vi "CalculateFeatures.vi"(7 "channels":T4[](array[typedef]), 8 "error in (no error)":errorcluster, 9 "pulse positions array":T3[](array[typedef]), 10 "waveforms":T2, 11 "Map":T1) -> (0 "error out":errorcluster, 5 "channels out":T4[](array[typedef]))   [LabVIEW 2017, in "AnalysisHelper.lvlib"]
uses:
  <vilib>/addons/InsightCM/Utilities/Analysis/Shared/AnalysisHelper.lvlib
  <vilib>/addons/InsightCM/Utilities/Analysis/Shared/controls/Channel.ctl
  <vilib>/addons/InsightCM/Utilities/Analysis/Shared/controls/SpeedType.ctl
  <vilib>/addons/InsightCM/Utilities/Analysis/Shared/controls/Feature.ctl
  <vilib>/addons/InsightCM/Utilities/Analysis/Shared/controls/AmplitudeScale.ctl
  <vilib>/addons/InsightCM/Utilities/Analysis/Shared/controls/PulsePositions.ctl
  <vilib>/addons/InsightCM/Utilities/DataAccessors/controls/wfmSGL_DVR.ctl
  <vilib>/addons/PointValueMap/controls/PointMap.ctl
  <vilib>/addons/InsightCM/Utilities/ChannelStatus/ChannelStatus.lvlib
  <vilib>/addons/PointValueMap/PointValueMap.lvlib
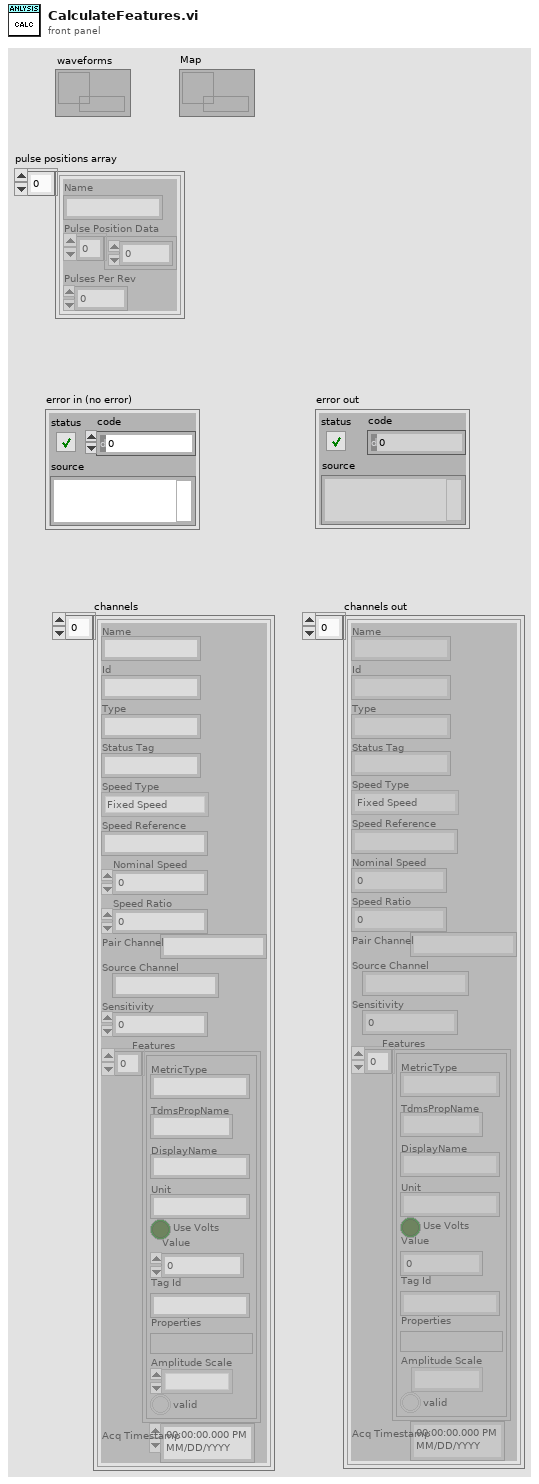
[diagram p1: front panel]
types:
  T1 = typedef "PointValueMap.lvlib/PointMap.ctl" = refnum<data-value>
  T2 = typedef "wfmSGL_DVR.ctl" = refnum<data-value>
  T3 = typedef "AnalysisHelper.lvlib/PulsePositions.ctl" = cluster{"Name":string, "Pulse Position Data":dbl[], "Pulses Per Rev":i32}
  T4 = typedef "AnalysisHelper.lvlib/Channel.ctl" = cluster{"Name":string, "Id":string, "Type":string, "Status Tag":string, "Speed Type":T5, "Speed Reference":string, "Nominal Speed":dbl, "Speed Ratio":dbl, "Pair Channel":string, "Source Channel":string, "Sensitivity":dbl, "Features":T6[], "Acq Timestamp":timestamp}
  T5 = typedef "AnalysisHelper.lvlib/SpeedType.ctl" = enum16{"Fixed Speed", "Tachometer", "From Map"}
  T6 = typedef "AnalysisHelper.lvlib/Feature.ctl" = cluster{"MetricType":string, "TdmsPropName":string, "DisplayName":string, "Unit":string, "Use Volts":bool, "Value":dbl, "Tag Id":string, "Properties":variant, "Amplitude Scale":T7, "valid":bool}
  T7 = typedef "AnalysisHelper.lvlib/AmplitudeScale.ctl" = enum16{"rms", "peak", "pk-pk"}
  T8 = typedef "AnalysisHelper.lvlib/LevelFeatures.ctl" = cluster{"RMS":dbl, "Peak":dbl, "Pk-Pk":dbl, "Derived Peak":dbl, "Crest Factor":dbl}
  T9 = typedef "AnalysisHelper.lvlib/MaxMinAvgFeatures.ctl" = cluster{"Max":dbl, "Min":dbl, "Avg":dbl}
  T10 = typedef "AnalysisHelper.lvlib/ConversionOp.ctl" = enum16{"none", "singleInt", "doubleInt", "singleDiff", "doubleDiff"}
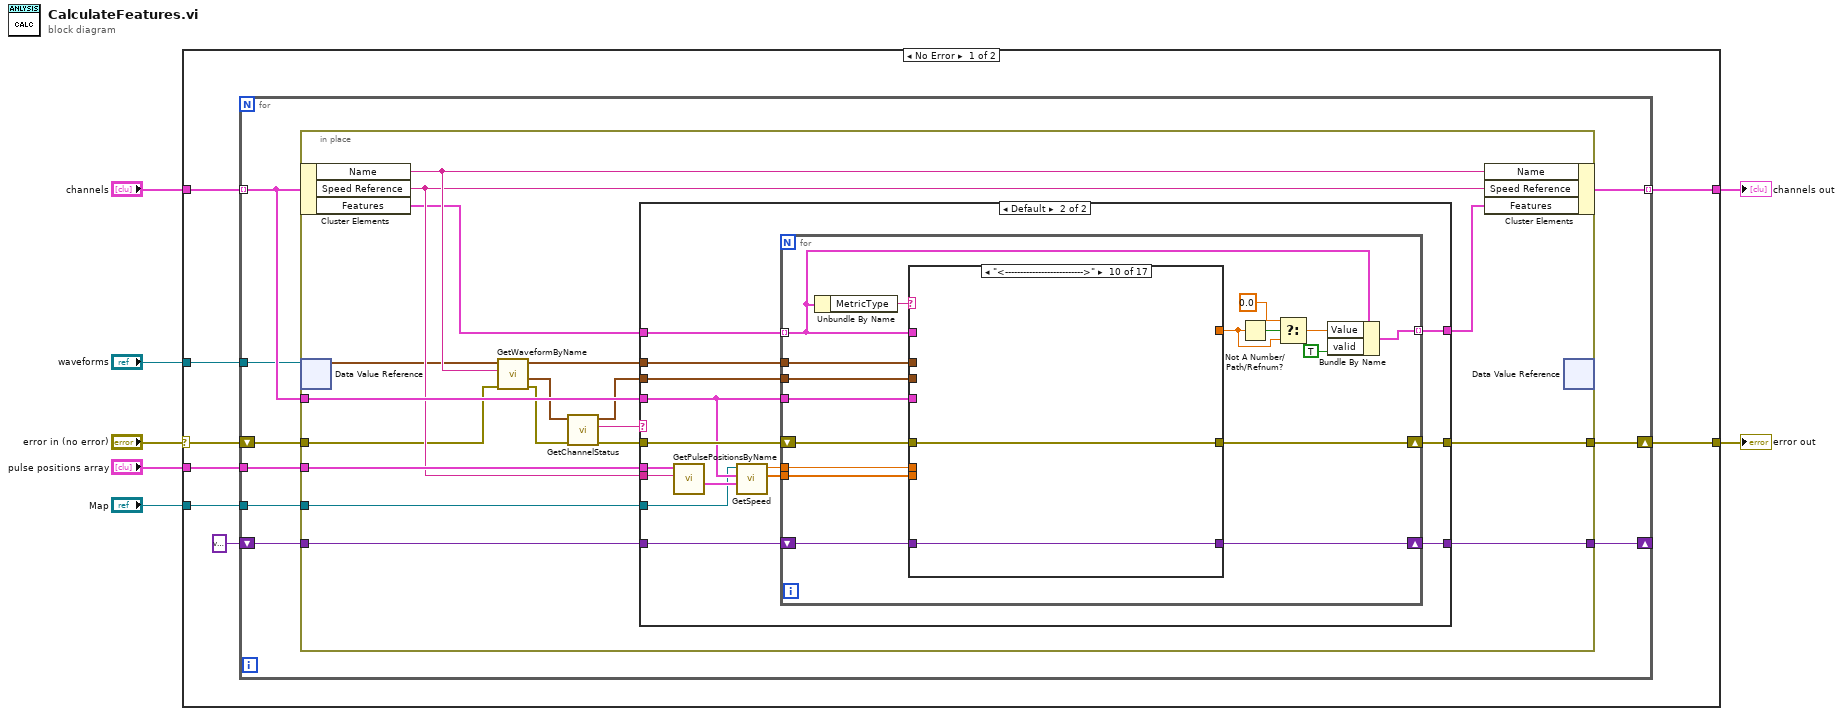
[diagram p0: block diagram]
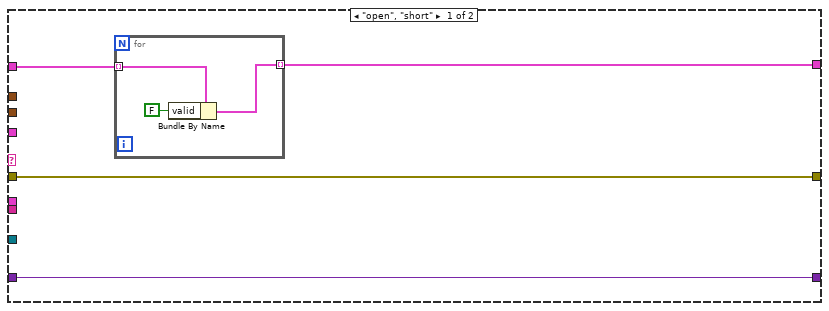
[diagram p2: hidden frame]
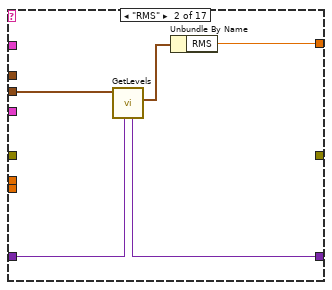
[diagram p4: hidden frame]
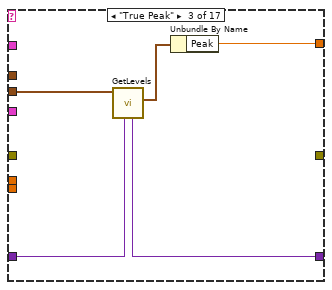
[diagram p5: hidden frame]
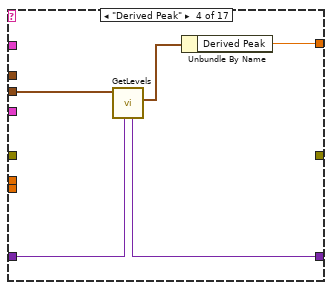
[diagram p6: hidden frame]
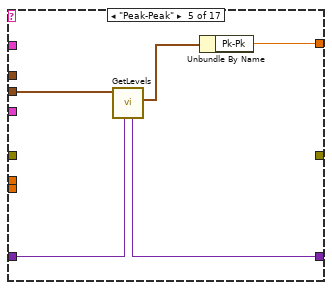
[diagram p7: hidden frame]
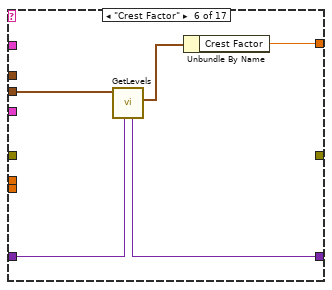
[diagram p8: hidden frame]
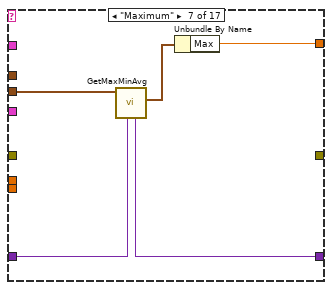
[diagram p9: hidden frame]
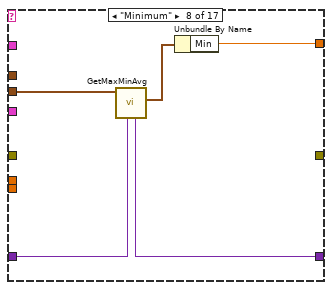
[diagram p10: hidden frame]
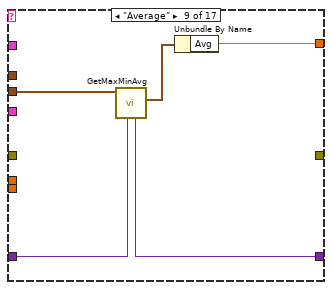
[diagram p11: hidden frame]
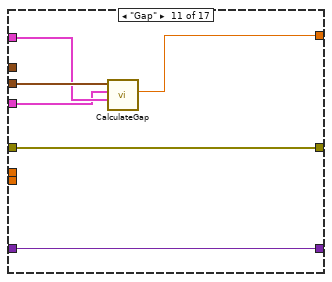
[diagram p12: hidden frame]
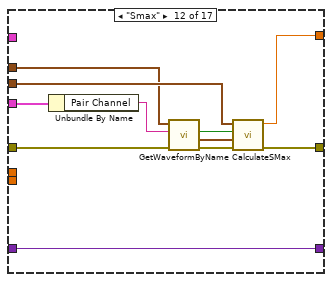
[diagram p13: hidden frame]
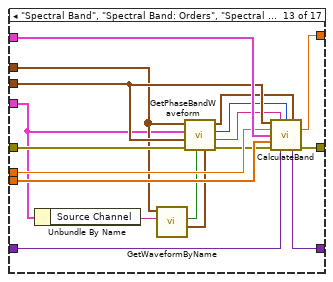
[diagram p14: hidden frame]
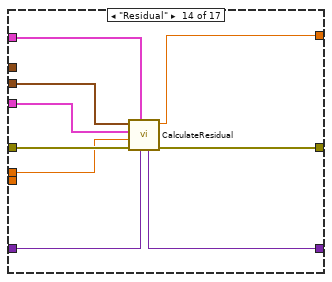
[diagram p15: hidden frame]
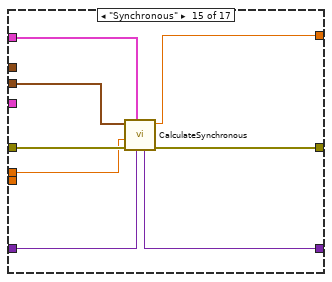
[diagram p16: hidden frame]
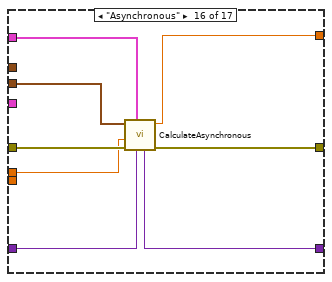
[diagram p17: hidden frame]
diagram:
  n1 = case shown="No Error" "error in (no error)" {
    selector: "error in (no error)" -> [w15 w188]
    tunnel: [w10 w188] -> w7
    tunnel: "channels" -> [w13 w189]
    tunnel: [w14 w189] -> w6
    tunnel: "pulse positions array" -> [w12 _]
    tunnel: "waveforms" -> [w9 _]
    tunnel: "Map" -> [w8 _]
    frame No Error {
      n2 = for {
        tunnel: w13 -> [w21] mode=indexing
        tunnel: [w24] -> w14 mode=indexing
        tunnel: w12 -> [w20]
        shift-right: [w18] -> _
        shift-left: variant -> [w19]
        shift-right: [w22] -> w10
        shift-left: w15 -> [w23]
        tunnel: w9 -> [w17]
        tunnel: w8 -> [w16]
        n3 = in-place {
          in-place-border: w23 -> [w34]
          in-place-border: [w42] -> w22
          in-place-border: w21 -> [w40]
          in-place-border: w20 -> [w37]
          in-place-border: w19 -> [w39]
          in-place-border: [w38] -> w18
          in-place-border: w16 -> [w25]
          n4 = in-place-cluster #1(w21) -> ("Name"=w41:string, "Speed Reference"=w35:string, "Features"=w33:T6[])
          n5 = in-place-dvr #2(w17) -> (w26:waveform(sgl)[])  [unwired: 1 out]
          n6 = call <vilib>:"GetWaveformByName.vi"("error in (no error)"=w34, "Channel Name"=w41, "Acq Waveforms"=w26) -> ("error out"=w31:errorcluster, "Waveform"=w28:waveform(sgl), "Acq Waveforms Out"=w36:waveform(sgl)[])  [unwired: 5 in, 1 out]
          n7 = call <vilib>:"GetChannelStatus.vi"("error in (no error)"=w31, "waveform in"=w28) -> ("error out"=w30:errorcluster, "channel status"=w29:string, "waveform out"=w27:waveform(sgl))  [unwired: 6 in, 1 out]
          n8 = case shown="Default" w29 {
            tunnel: [w44 w64] -> w32
            tunnel: w30 -> [w43 w63]
            tunnel: w33 -> [w45 w62]
            tunnel: w40 -> [_ w53]
            tunnel: w36 -> [_ w61]
            tunnel: w27 -> [_ w60]
            tunnel: [w43 w57] -> w42
            tunnel: w39 -> [w46 w59]
            tunnel: [w46 w58] -> w38
            tunnel: w37 -> [_ w56]
            tunnel: w35 -> [_ w55]
            tunnel: w25 -> [_ w50]
            frame "open", "short" {
              n9 = for {
                tunnel: w45 -> [w49] mode=indexing
                tunnel: [w47] -> w44 mode=indexing
                n10 = Bundle By Name(cluster=w49, "valid"=FALSE) -> (w47:T6)
              }
            }
            frame Default {
              n11 = call <vilib>:"GetPulsePositionsByName.vi"("Channel Name"=w55, "Pulse Positions Array"=w56) -> ("Pulse Positions"=w54:T3)  [unwired: 6 in, 3 out]
              n12 = call <vilib>:"GetSpeed.vi"("pulse positions"=w54, "channel"=w53, "Map"=w50) -> ("pulse position data"=w52:dbl[], "speed (RPM)"=w51:dbl)  [unwired: 7 in]
              n13 = for {
                tunnel: w62 -> [w75] mode=indexing
                tunnel: w60 -> [w80]
                tunnel: [w81] -> w64 mode=indexing
                tunnel: w61 -> [w77]
                tunnel: w53 -> [w76]
                shift-right: [w72] -> w58
                shift-left: w59 -> [w73]
                shift-right: [w78] -> w57
                shift-left: w63 -> [w79]
                tunnel: w52 -> [w70]
                tunnel: w51 -> [w71]
                n14 = Unbundle By Name(w75) -> ("MetricType"=w74:string)
                n15 = case shown="\"<-------------------------->\"" w74 {
                  tunnel: [w82 w84 w89 w94 w99 w104 w111 w116 w121 _ w130 w141 w159 w166 w171 w178 _] -> w67
                  tunnel: w80 -> [_ w87 w92 w97 w102 w107 w112 w117 w122 _ w131 w140 w153 w168 w177 w184 _]
                  tunnel: w79 -> [_ _ _ _ _ _ _ _ _ w124 w129 w135 w152 w169 w176 w183 w186]
                  tunnel: [_ _ _ _ _ _ _ _ _ w124 w129 w142 w160 w167 w175 w182 w186] -> w78
                  tunnel: w77 -> [_ _ _ _ _ _ _ _ _ _ _ w136 w147 _ _ _ _]
                  tunnel: w76 -> [_ _ _ _ _ _ _ _ _ _ w127 w137 w146 w165 _ _ _]
                  tunnel: w75 -> [_ _ _ _ _ _ _ _ _ _ w128 _ w158 w164 w170 w185 _]
                  tunnel: w73 -> [w83 w86 w91 w96 w101 w106 w110 w115 w120 w125 w126 w139 w156 w162 w174 w181 w187]
                  tunnel: [w83 w85 w90 w95 w100 w105 w109 w114 w119 w125 w126 w139 w157 w163 w173 w180 w187] -> w72
                  tunnel: w71 -> [w82 _ _ _ _ _ _ _ _ _ _ _ w154 w161 w172 w179 _]
                  tunnel: w70 -> [_ _ _ _ _ _ _ _ _ _ _ _ w155 _ _ _ _]
                  frame "Speed" {
                  }
                  frame "RMS" {
                    n16 = call <vilib>:"GetLevels.vi"("calc cache"=w86, "waveform"=w87) -> ("levels"=w88:T8, "calc cache out"=w85:variant)  [unwired: 8 in]
                    n17 = Unbundle By Name(w88) -> ("RMS"=w84:dbl)
                  }
                  frame "True Peak" {
                    n18 = call <vilib>:"GetLevels.vi"("calc cache"=w91, "waveform"=w92) -> ("levels"=w93:T8, "calc cache out"=w90:variant)  [unwired: 8 in]
                    n19 = Unbundle By Name(w93) -> ("Peak"=w89:dbl)
                  }
                  frame "Derived Peak" {
                    n20 = call <vilib>:"GetLevels.vi"("calc cache"=w96, "waveform"=w97) -> ("levels"=w98:T8, "calc cache out"=w95:variant)  [unwired: 8 in]
                    n21 = Unbundle By Name(w98) -> ("Derived Peak"=w94:dbl)
                  }
                  frame "Peak-Peak" {
                    n22 = call <vilib>:"GetLevels.vi"("calc cache"=w101, "waveform"=w102) -> ("levels"=w103:T8, "calc cache out"=w100:variant)  [unwired: 8 in]
                    n23 = Unbundle By Name(w103) -> ("Pk-Pk"=w99:dbl)
                  }
                  frame "Crest Factor" {
                    n24 = call <vilib>:"GetLevels.vi"("calc cache"=w106, "waveform"=w107) -> ("levels"=w108:T8, "calc cache out"=w105:variant)  [unwired: 8 in]
                    n25 = Unbundle By Name(w108) -> ("Crest Factor"=w104:dbl)
                  }
                  frame "Maximum" {
                    n26 = call <vilib>:"GetMaxMinAvg.vi"("calc cache"=w110, "waveform"=w112) -> ("MaxMinAvg"=w113:T9, "calc cache out"=w109:variant)  [unwired: 8 in]
                    n27 = Unbundle By Name(w113) -> ("Max"=w111:dbl)
                  }
                  frame "Minimum" {
                    n28 = call <vilib>:"GetMaxMinAvg.vi"("calc cache"=w115, "waveform"=w117) -> ("MaxMinAvg"=w118:T9, "calc cache out"=w114:variant)  [unwired: 8 in]
                    n29 = Unbundle By Name(w118) -> ("Min"=w116:dbl)
                  }
                  frame "Average" {
                    n30 = call <vilib>:"GetMaxMinAvg.vi"("calc cache"=w120, "waveform"=w122) -> ("MaxMinAvg"=w123:T9, "calc cache out"=w119:variant)  [unwired: 8 in]
                    n31 = Unbundle By Name(w123) -> ("Avg"=w121:dbl)
                  }
                  frame "<-------------------------->" {
                  }
                  frame "Gap" {
                    n32 = call <vilib>:"CalculateGap.vi"("feature"=w128, "channel"=w127, "waveform data"=w131) -> ("gap"=w130:dbl)  [unwired: 8 in]
                  }
                  frame "Smax" {
                    n33 = Unbundle By Name(w137) -> ("Pair Channel"=w138:string)
                    n34 = call <vilib>:"GetWaveformByName.vi"("error in (no error)"=w135, "Channel Name"=w138, "Acq Waveforms"=w136) -> ("error out"=w134:errorcluster, "Waveform"=w132:waveform(sgl), "Found?"=w133:bool)  [unwired: 5 in, 1 out]
                    n35 = call <vilib>:"CalculateSMax.vi"("error in (no error)"=w134, "pair waveform"=w132, "pair waveform found"=w133, "Waveform"=w140) -> ("error out"=w142:errorcluster, "Smax"=w141:dbl)  [unwired: 6 in]
                  }
                  frame "Spectral Band", "Spectral Band: Orders", "Spectral Band: Phase" {
                    n36 = Unbundle By Name(w146) -> ("Source Channel"=w145:string)
                    n37 = call <vilib>:"GetWaveformByName.vi"("Channel Name"=w145, "Acq Waveforms"=w147) -> ("Waveform"=w143:waveform(sgl), "Found?"=w144:bool)  [unwired: 6 in, 2 out]
                    n38 = call <vilib>:"GetPhaseBandWaveform.vi"("source channel wfm"=w143, "source channel wfm found"=w144, "error in (no error)"=w152, "waveform"=w153, "channel"=w146, "all waveforms"=w147) -> ("error out"=w151:errorcluster, "channel name of waveform to use in phase band calculation"=w148:string, "conversion op"=w149:T10, "waveform to use in phase band calculation"=w150:waveform(sgl))  [unwired: 2 in]
                    n39 = call <vilib>:"CalculateBand.vi"("waveform"=w153, "channel name of waveform to use in phase band calculation"=w148, "conversion op"=w149, "waveform to use in phase band calculation"=w150, "speed [RPM]"=w154, "feature"=w158, "pulse positions"=w155, "error in (no error)"=w151, "calc cache"=w156) -> ("band value"=w159:dbl, "calc cache out"=w157:variant, "error out"=w160:errorcluster)  [unwired: 4 in]
                  }
                  frame "Residual" {
                    n40 = call <vilib>:"CalculateResidual.vi"("calc cache"=w162, "Feature"=w164, "error in (no error)"=w169, "Speed (RPM)"=w161, "Channel"=w165, "Data"=w168) -> ("error out"=w167:errorcluster, "Residual [EU RMS]"=w166:dbl, "calc cache out"=w163:variant)  [unwired: 3 in]
                  }
                  frame "Synchronous" {
                    n41 = call <vilib>:"CalculateSynchronous.vi"("calc cache"=w174, "Feature"=w170, "error in (no error)"=w176, "Speed (RPM)"=w172, "Data"=w177) -> ("error out"=w175:errorcluster, "Synchronous [EU RMS]"=w171:dbl, "calc cache out"=w173:variant)  [unwired: 4 in]
                  }
                  frame "Asynchronous" {
                    n42 = call <vilib>:"CalculateAsynchronous.vi"("calc cache"=w181, "Feature"=w185, "error in (no error)"=w183, "Speed (RPM)"=w179, "Data"=w184) -> ("error out"=w182:errorcluster, "Asynchronous [EU RMS]"=w178:dbl, "calc cache out"=w180:variant)  [unwired: 4 in]
                  }
                  frame Default {
                  }
                }
                n43 = Not A Number/Path/Refnum?(number/path/refnum=w67) -> (NaN/Path/Refnum?=w66:bool)
                n44 = Select(t=0.0, s=w66, f=w67) -> (s? t:f=w69:dbl)
                n45 = Bundle By Name(cluster=w75, "Value"=w69, "valid"=TRUE) -> (w81:T6)
              }
            }
          }
          n46 = in-place-cluster #1("Name"=w41, "Speed Reference"=w35, "Features"=w32) -> (w24:T4)
          n47 = in-place-dvr #2() -> ()  [unwired: 1 in, 2 out]
        }
      }
    }
    frame Error {
    }
  }
  "error out" <- w7
  "channels out" <- w6
